vi "PQ test 1.vi"() -> ()   [LabVIEW 2015, in "PQ Result.lvclass"]
uses:
  Result/PQ Result.lvclass
  Result/PQ Result.lvclass/PQ Result.ctl
  Result/Write Next Row (First Column).vi
  Result/Number of Rows.vi
  Result/Get Column String.vi
  Result/Get Column DBL.vi
  Connection/PQ Connection.lvclass
panel:
  out "Array":T1(array[cluster]) {"Get:Get DBL" format="%#_16g"}
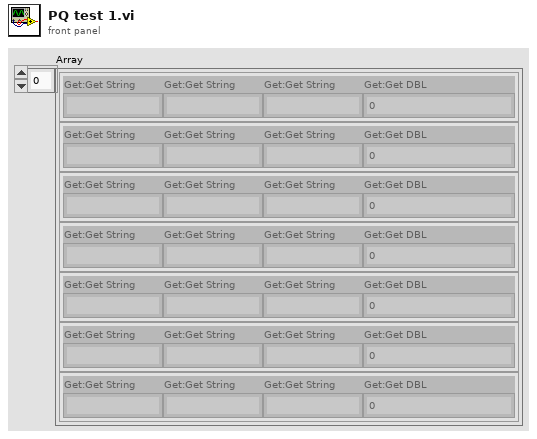
[diagram p1: front panel]
types:
  T1 = cluster{"Get:Get String":string, "Get:Get String":string, "Get:Get String":string, "Get:Get DBL":dbl}[]
  T2 = cluster{"Get:Get String":string, "Get:Get String":string, "Get:Get String":string, "Get:Get DBL":dbl}
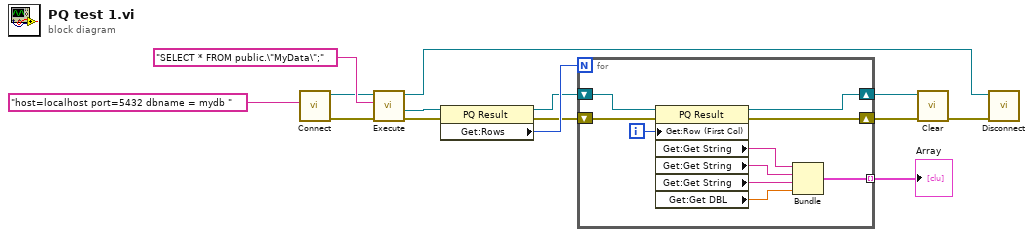
[diagram p0: block diagram]
diagram:
  n1 = call "Connect.vi"("conninfo"="host=localhost port=5432 dbname = mydb ") -> ("error out"=w2:errorcluster, "PQ Connection out"=w11:refnum<class "PQ Connection.lvclass">)  [unwired: 8 in, 1 out]
  n2 = call "Execute.vi"("error in (no error)"=w2, "command"="SELECT * FROM public.\"MyData\";", "PQ Connection in"=w11) -> ("error out"=w3:errorcluster, "PQ Result  out"=w6:refnum<class "PQ Result.lvclass">, "PQ Connection out"=w10:refnum<class "PQ Connection.lvclass">)  [unwired: 5 in, 1 out]
  n3 = property class="PQ Result"(reference=w6, error in=w3) -> (reference out=w8:refnum<class "PQ Result.lvclass">, error out=w7:errorcluster, "Get:Rows"=w9:i32)
  n4 = for {
    N: w9 -> [_]
    shift-right: [w24] -> w5
    shift-left: w8 -> [w17]
    shift-right: [w23] -> w1
    shift-left: w7 -> [w16]
    tunnel: [w18] -> w4 mode=indexing
    i -> [w15]
    n5 = property class="PQ Result"(reference=w17, error in=w16, "Get:Row (First Col)"=w15) -> (reference out=w24:refnum<class "PQ Result.lvclass">, error out=w23:errorcluster, "Get:Get String"=w22:string, "Get:Get String"=w21:string, "Get:Get String"=w20:string, "Get:Get DBL"=w19:dbl)
    n6 = Bundle("Get:Get String"=w22, "Get:Get String"=w21, "Get:Get String"=w20, "Get:Get DBL"=w19) -> (w18:T2)  [unwired: 1 in]
  }
  "Array" <- w4
  n7 = call "Clear.vi"("error in (no error)"=w1, "PQ Result  in"=w5) -> ("error out"=w12:errorcluster)  [unwired: 9 in]
  n8 = call "Disconnect.vi"("error in (no error)"=w12, "PQ Connection in"=w10) -> ()  [unwired: 9 in, 1 out]
